vi "PipBoy_NotifyChangeContextMenu.vi"(8 "error in (no error)":errorcluster, 10 "LabVIEWEvent":T1, 11 "PipBoyDataIn":T3) -> (0 "error out":errorcluster, 3 "PipBoyDataOut":T3)   [LabVIEW 2014]
uses:
  ctls/PipBoy_PipBoyData.ctl
  ctls/PipBoy_ProcComm.ctl
  System.Windows.Forms
  ctls/PipBoy_PipBoyCommand.ctl
  ctls/PipBoy_Message.ctl
  modules/support/Message Queue/All Message Queues.ctl
  modules/support/Message Queue/Message Cluster.ctl
  ctls/PipBoy_FileConf.ctl
  ctls/PipBoy_PicComm.ctl
  ctls/PipBoy_GeneralParams.ctl
  ctls/PipBoy_Pages.ctl
  ctls/PipBoy_LabVIEWEvent.ctl
  ctls/PipBoy_DetectionType.ctl
  <userlib>/NotifyIcon/TypeDefs/NotifyIcon Event Registration Actions.ctl
  <userlib>/NotifyIcon/TypeDefs/NotifyIcon Events.ctl
  modules/support/Message Queue/Message Queue.lvlib
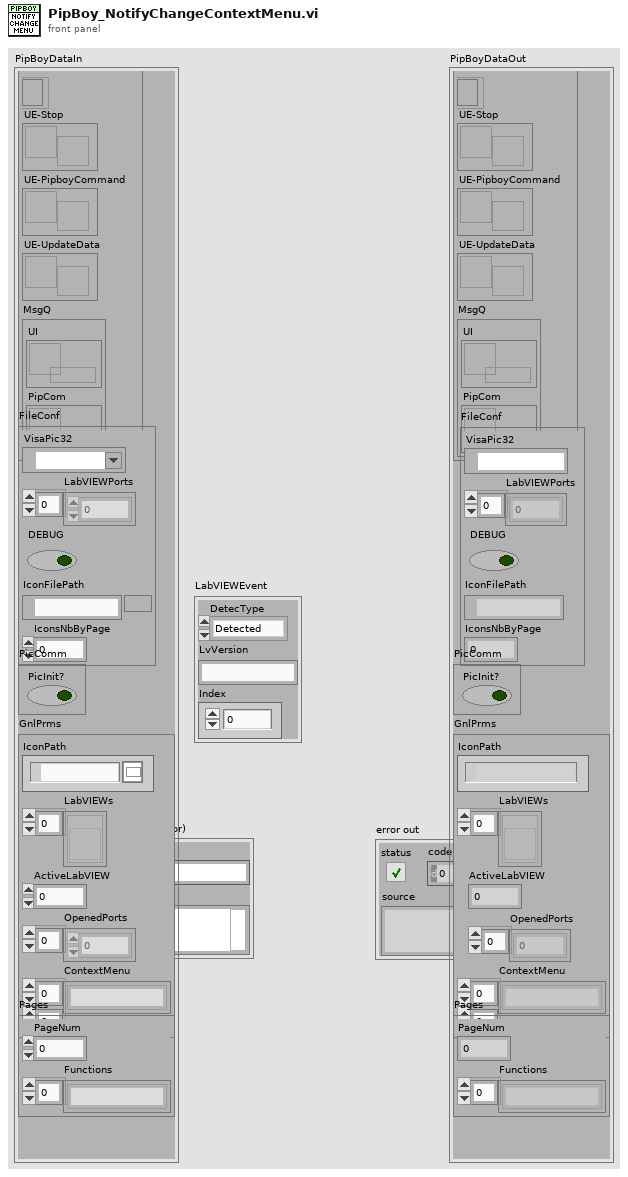
[diagram p1: front panel]
types:
  T1 = typedef "PipBoy_LabVIEWEvent.ctl" = cluster{"DetecType":T2, "LvVersion":string, "Index":i32}
  T2 = typedef "PipBoy_DetectionType.ctl" = enum16{"Detected", "Lost"}
  T3 = typedef "PipBoy_PipBoyData.ctl" = cluster{"ProcComm":T4, "FileConf":T6, "PicComm":T7, "GnlPrms":T8, "Pages":T9}
  T4 = typedef "PipBoy_ProcComm.ctl" = cluster{"NotifyIconRef":refnum<k24>, "UE-Stop":refnum<user-event>, "UE-PipboyCommand":refnum<user-event>, "UE-UpdateData":refnum<user-event>, "MsgQ":T5}
  T5 = typedef "Message Queue.lvlib/All Message Queues.ctl" = cluster{"UI":refnum<queue>, "PipCom":refnum<queue>}
  T6 = typedef "PipBoy_FileConf.ctl" = cluster{"VisaPic32":refnum<visa-resource-name>, "LabVIEWPorts":u16[], "DEBUG":bool, "IconFilePath":path, "IconsNbByPage":i32}
  T7 = typedef "PipBoy_PicComm.ctl" = cluster{"PicInit?":bool}
  T8 = typedef "PipBoy_GeneralParams.ctl" = cluster{"IconPath":path, "LabVIEWs":refnum<vi>[], "ActiveLabVIEW":i32, "OpenedPorts":u16[], "ContextMenu":string[][]}
  T9 = typedef "PipBoy_Pages.ctl" = cluster{"PageNum":i32, "Functions":string[]}
  T10 = typedef "NotifyIcon Event Registration Actions.ctl" = enum16{"Initial Event Registration", "Add to Event Registration", "Destroy Events and Re-register"}
  T11 = typedef "PipBoy_Message.ctl" = cluster{"Name":string, "Data":variant}
  T12 = typedef "NotifyIcon Events.ctl" = enum16{"BalloonTipClicked", "BalloonTipClosed", "BalloonTipShown", "Click", "Disposed", "DoubleClick", "MouseClick", "MouseDoubleClick", "MouseDown", "MouseMove", "MouseUp", "MenuItemClick", "MenuItemSelect"}
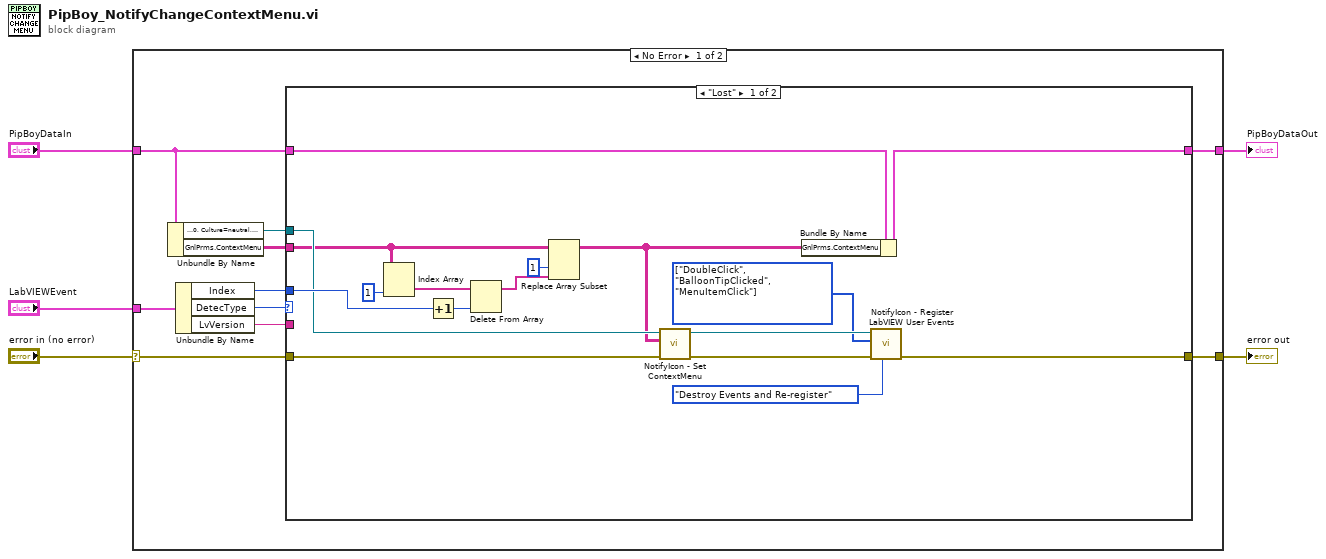
[diagram p0: block diagram]
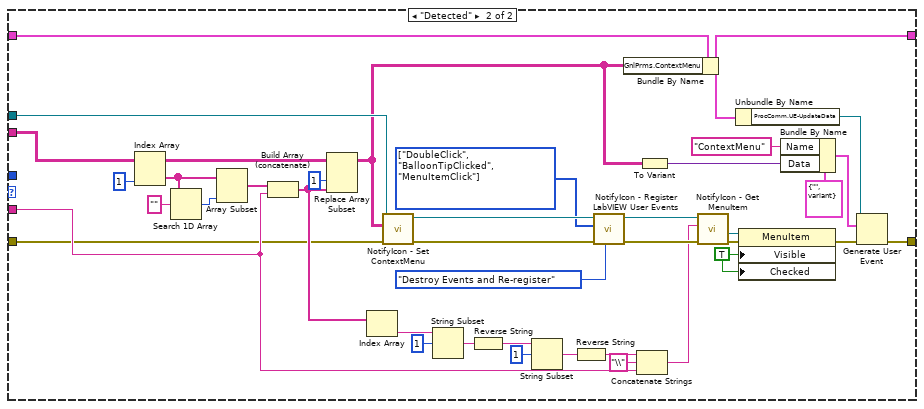
[diagram p2: hidden frame]
diagram:
  n1 = case shown="No Error" "error in (no error)" {
    selector: "error in (no error)" -> [w13 w73]
    tunnel: [w14 w73] -> w4
    tunnel: [w11 w72] -> w2
    tunnel: "PipBoyDataIn" -> [w12 w72]
    tunnel: "LabVIEWEvent" -> [w10 _]
    frame No Error {
      n2 = Unbundle By Name(w12) -> ("ProcComm.NotifyIconRef"=w15:refnum<k24>, "GnlPrms.ContextMenu"=w7:string[][])
      n3 = Unbundle By Name(w10) -> ("Index"=w6:i32, "DetecType"=w8:T2, "LvVersion"=w9:string)
      n4 = case shown="\"Lost\"" w8 {
        tunnel: w15 -> [w19 w67]
        tunnel: [w20 w41] -> w14
        tunnel: w13 -> [w21 w42]
        tunnel: w7 -> [w17 w59]
        tunnel: w12 -> [w32 w60]
        tunnel: [w31 w39] -> w11
        tunnel: w9 -> [_ w43]
        tunnel: w6 -> [w28 _]
        frame "Lost" {
          w22 = T12[] [enum."DoubleClick", enum."BalloonTipClicked", enum."MenuItemClick"] items=["BalloonTipClicked", "BalloonTipClosed", "BalloonTipShown", "Click", "Disposed", "DoubleClick", "MouseClick", "MouseDoubleClick", "MouseDown", "MouseMove", "MouseUp", "MenuItemClick", "MenuItemSelect"] ("Events to register")
          n5 = Index Array(array=w17, index (col)=1 ("disabled index (col)")) -> (element=w29:string[])  [unwired: 1 in]
          n6 = Increment(x=w28) -> (x+1=w16:i32)
          n7 = Delete From Array(array=w29, index=w16) -> (array with subset deleted=w27:string[])  [unwired: 1 in, 1 out]
          n8 = Replace Array Subset(array=w17, new element=w27, index (col)=1 ("disabled index (col)")) -> (w18:string[][])  [unwired: 1 in]
          n9 = call <userlib>:"NotifyIcon - Set ContextMenu.vi"("error in"=w21, "Context Menu"=w18, "NotifyIcon reference in"=w19) -> ("error out"=w24:errorcluster, "NotifyIcon reference out"=w25:refnum<k24>)  [unwired: 7 in]
          n10 = Bundle By Name(cluster=w32, "GnlPrms.ContextMenu"=w18) -> (w31:T3)
          n11 = call <userlib>:"NotifyIcon - Register LabVIEW User Events.vi"("Action"=NotifyIcon_Event_Registration_Actions."Destroy Events and Re-register", "error in"=w24, "Events to register"=w22, "NotifyIcon reference in"=w25) -> ("error out"=w20:errorcluster)  [unwired: 5 in, 2 out]
        }
        frame "Detected" {
          w51 = TRUE ("Visible")
          w68 = T12[] [enum."DoubleClick", enum."BalloonTipClicked", enum."MenuItemClick"] items=["BalloonTipClicked", "BalloonTipClosed", "BalloonTipShown", "Click", "Disposed", "DoubleClick", "MouseClick", "MouseDoubleClick", "MouseDown", "MouseMove", "MouseUp", "MenuItemClick", "MenuItemSelect"] ("Events to register")
          n12 = Index Array(array=w59, index (col)=1 ("disabled index (col)")) -> (element=w64:string[])  [unwired: 1 in]
          n13 = Search 1D Array(1D array=w64, element="") -> (index of element=w63:i32)  [unwired: 1 in]
          n14 = Array Subset(array=w64, length=w63) -> (w62:string[])  [unwired: 1 in]
          n15 = Build Array (concatenate)(w62, w43) -> (w56:string[])
          n16 = Replace Array Subset(array=w59, new element=w56, index (col)=1 ("disabled index (col)")) -> (w37:string[][])  [unwired: 1 in]
          n17 = Index Array(array=w56) -> (element=w45:string)  [unwired: 1 in]
          n18 = call <userlib>:"NotifyIcon - Set ContextMenu.vi"("error in"=w42, "Context Menu"=w37, "NotifyIcon reference in"=w67) -> ("error out"=w70:errorcluster, "NotifyIcon reference out"=w71:refnum<k24>)  [unwired: 7 in]
          n19 = String Subset(string=w45, offset (0)=1) -> (substring=w49:string)  [unwired: 1 in]
          n20 = Reverse String(1:w49) -> (0:w48:string)
          n21 = String Subset(string=w48, offset (0)=1) -> (substring=w46:string)  [unwired: 1 in]
          n22 = Reverse String(1:w46) -> (0:w44:string)
          n23 = call <userlib>:"NotifyIcon - Register LabVIEW User Events.vi"("Action"=NotifyIcon_Event_Registration_Actions."Destroy Events and Re-register", "error in"=w70, "Events to register"=w68, "NotifyIcon reference in"=w71) -> ("error out"=w58:errorcluster, "NotifyIcon reference out"=w57:refnum<k24>)  [unwired: 5 in, 1 out]
          n24 = Bundle By Name(cluster=w60, "GnlPrms.ContextMenu"=w37) -> (w39:T3)
          n25 = Concatenate Strings(w44, "\\" ("element"), w43) -> (w54:string)
          n26 = To Variant(anything=w37) -> (Variant=w35:variant)
          n27 = call <userlib>:"NotifyIcon - Get MenuItem.vi"("error in"=w58, "Context MenuItem"=w54, "NotifyIcon reference in"=w57) -> ("error out"=w53:errorcluster, "MenuItem reference"=w52:refnum<k24>)  [unwired: 6 in, 1 out]
          n28 = Unbundle By Name(w39) -> ("ProcComm.UE-UpdateData"=w38:refnum<user-event>)
          n29 = property class="MenuItem"(reference=w52, error in=w53, "Visible"=w51, "Checked"=w51) -> (error out=w40:errorcluster)  [unwired: 1 out]
          n30 = Bundle By Name(cluster=T11 {"Name"="", "Data"=variant} ("event data"), "Name"="ContextMenu", "Data"=w35) -> (w34:T11)
          n31 = Generate User Event(user event=w38, event data cluster=w34, error in=w40) -> (error out=w41:errorcluster)  [unwired: 1 in, 1 out]
        }
      }
    }
    frame Error {
    }
  }
  "error out" <- w4
  "PipBoyDataOut" <- w2
